vi "JSON Formater.vi"(4 "Disable LabVIEW Extensions":bool, 6 "Pretty Print":bool, 7 "Comment out unparsable lines":bool, 8 "error in":errorcluster, 10 "Offset":i32, 11 "JSON":string) -> (0 "error OUT":errorcluster, 2 "Rest of Input String":string, 3 "<JSON>":string)   [LabVIEW 2020, in "JSONtext.lvlib"]
uses:
  <vilib>/JDP Science/JSONtext/JSONtext.lvlib
  <vilib>/JDP Science/JSONtext/Parsing/Parsing State.ctl
  <vilib>/JDP Science/JSONtext/Parsing/Token Type.ctl
panel:
  in  "Pretty Print Levels":i32=9
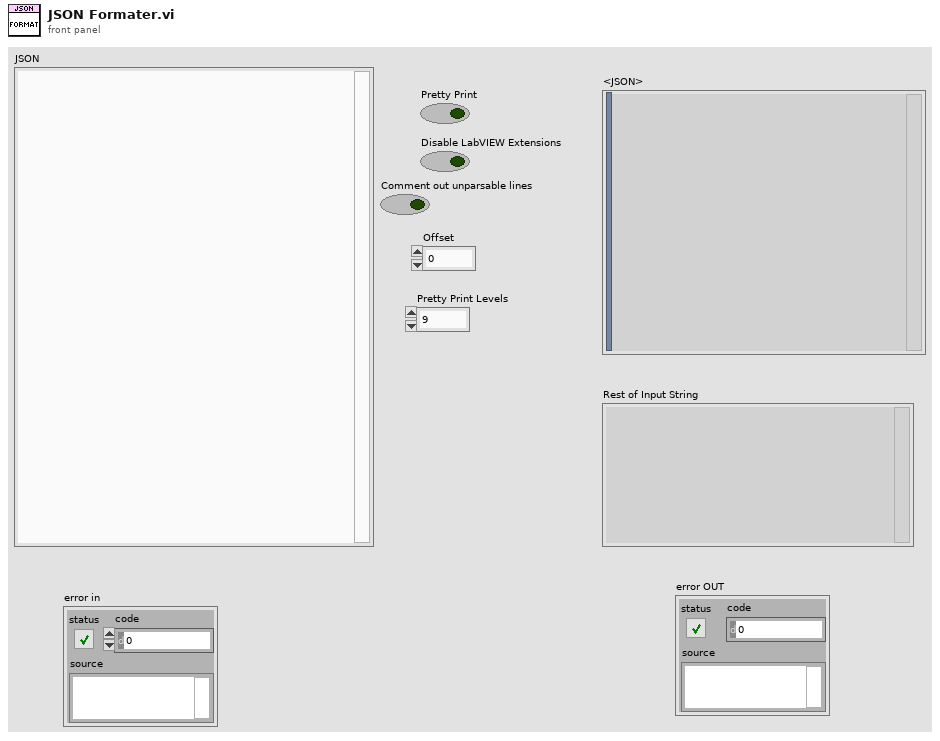
[diagram p1: front panel]
types:
  T1 = typedef "JSONtext.lvlib/Parsing State.ctl" = enum16{"Parser Error", "Object", "Array", "String", "Number/Other", "Leading Whitespace", "Object end", "Array end", "Value end"}
  T2 = typedef "JSONtext.lvlib/Token Type.ctl" = enum16{"Error", "Scalar", "comma", "colon", "Comment", "Down", "Up", "Line End", "Make Null", "Inline Comment", "Ignore", "junk line"}
  T3 = cluster{"Offset of first non-whitespace":i32, "Offset of first non-whitespace":i32, T2}
  T4 = typedef "JSONtext.lvlib/Token.ctl" = cluster{"Start":i32, "End":i32, "Type":T2}
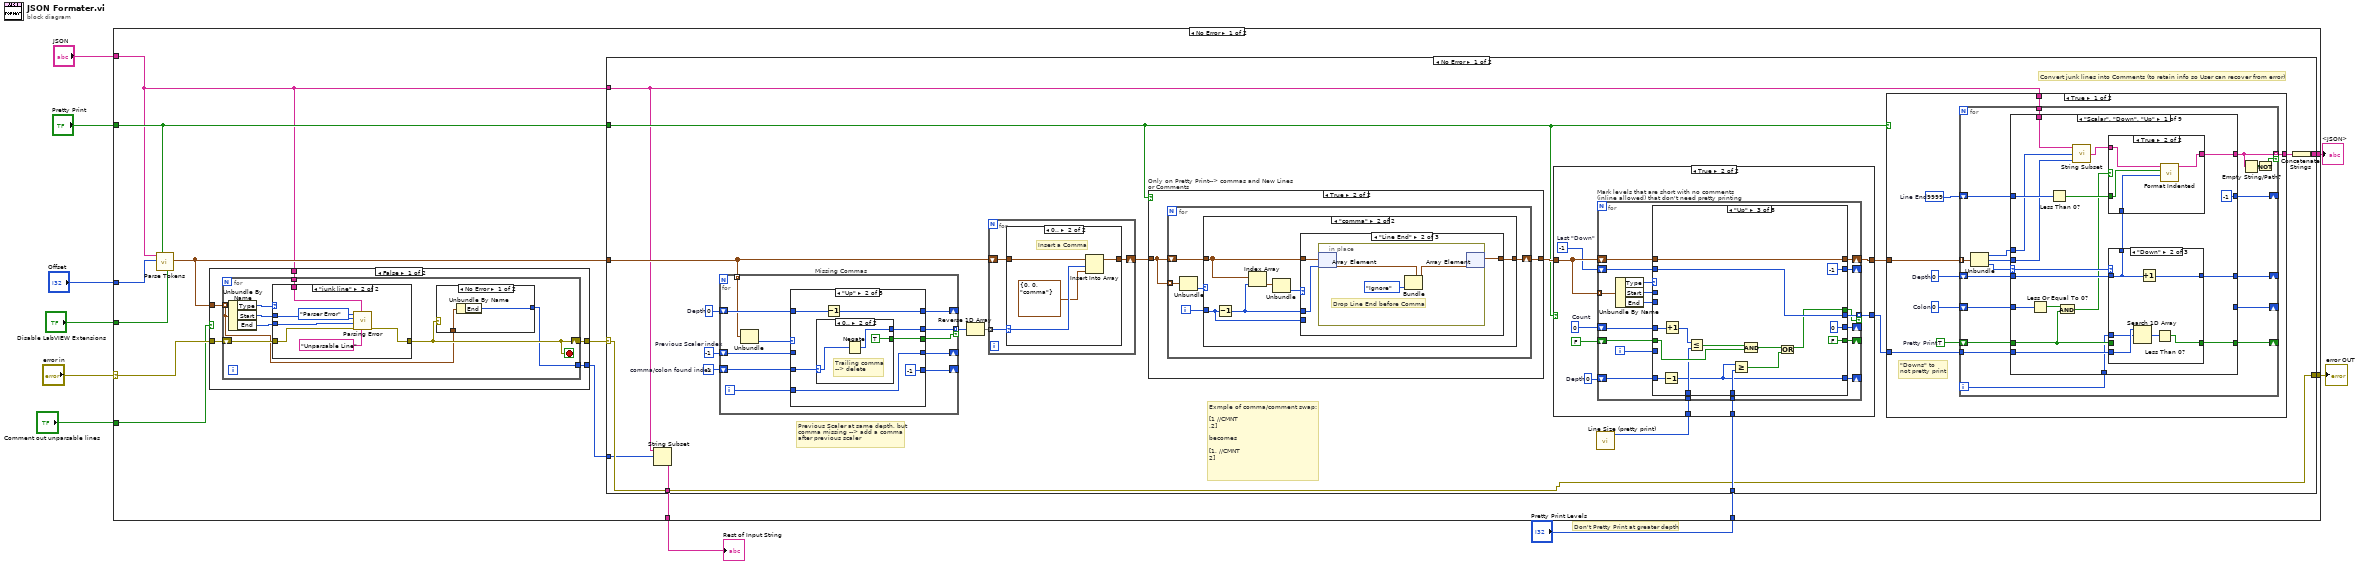
[diagram p0: block diagram]
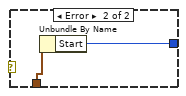
[diagram p2: hidden frame]
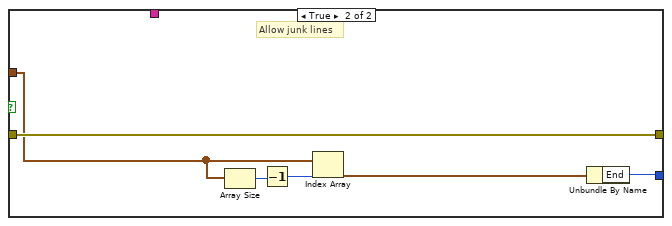
[diagram p4: hidden frame]
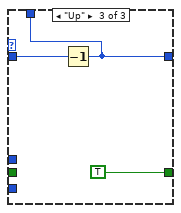
[diagram p7: hidden frame]
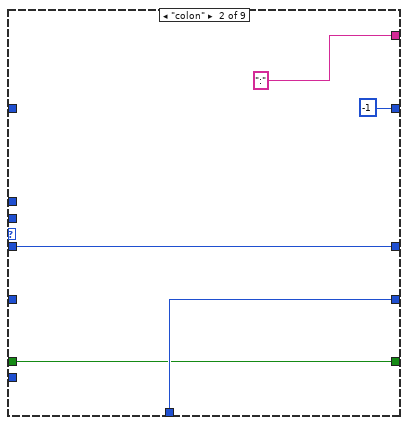
[diagram p8: hidden frame]
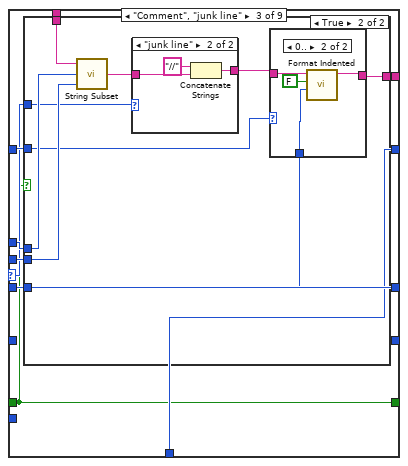
[diagram p9: hidden frame]
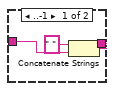
[diagram p12: hidden frame]
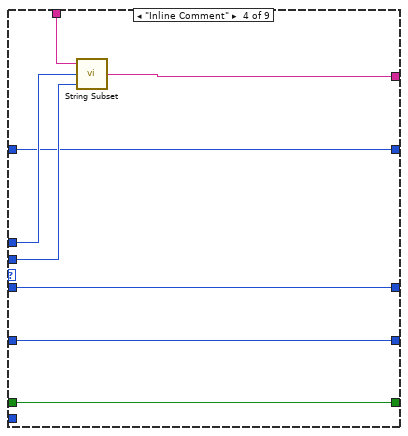
[diagram p13: hidden frame]
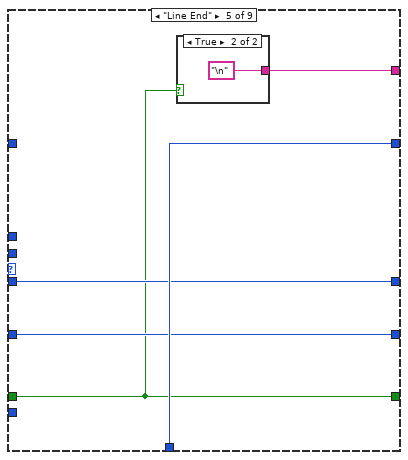
[diagram p14: hidden frame]
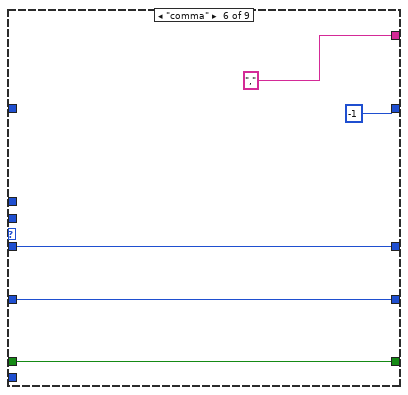
[diagram p16: hidden frame]
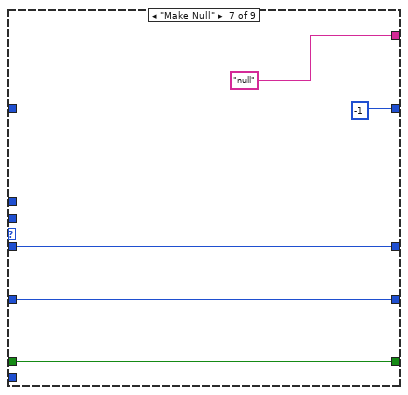
[diagram p17: hidden frame]
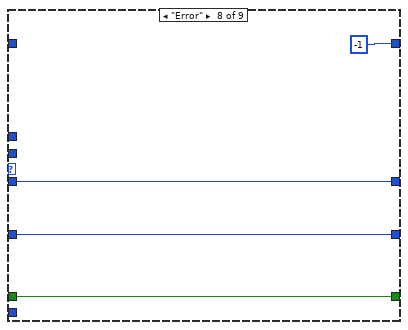
[diagram p18: hidden frame]
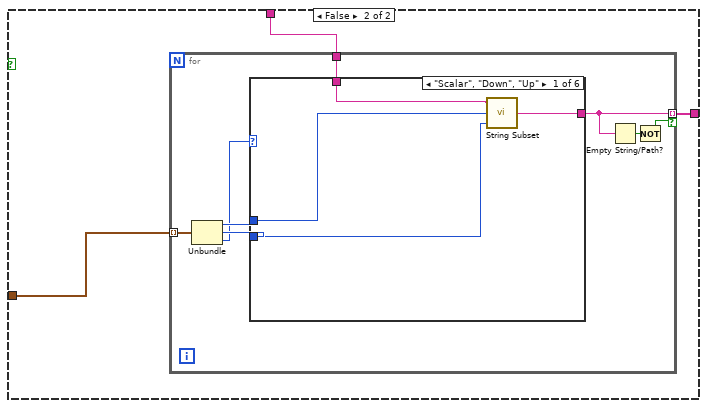
[diagram p20: hidden frame]
diagram:
  # "Don't Pretty Print at greater depth"
  n1 = case shown="No Error" "error in" {
    selector: "error in" -> [w18 w394]
    tunnel: [w23 _] -> w10
    tunnel: "Disable LabVIEW Extensions" -> [w22 _]
    tunnel: "Offset" -> [w21 _]
    tunnel: "Pretty Print" -> [w20 _]
    tunnel: "JSON" -> [w13 w393]
    tunnel: "Pretty Print Levels" -> [w17 _]
    tunnel: [w15 w394] -> w3
    tunnel: "Comment out unparsable lines" -> [w14 _]
    tunnel: [w11 w393] -> w1
    frame No Error {
      n2 = call <vilib>:"Parse Tokens.vi"("Disable LabVIEW Extensions"=w22, "Pretty Print"=w20, "Offset"=w21, "JSON"=w13) -> ("Tokens"=w19:T4[])  [unwired: 7 in]
      n3 = case shown="False" w14 {
        tunnel: w19 -> [w28 w53]
        tunnel: w13 -> [w27 _]
        tunnel: w18 -> [w26 w54]
        tunnel: [w25 w54] -> w16
        tunnel: [w24 w49] -> w12
        frame False {
          n4 = for {
            tunnel: w28 -> [w30] mode=indexing
            tunnel: w27 -> [w35]
            shift-right: [w31] -> w25
            shift-left: w26 -> [w34]
            tunnel: [w29] -> w24
            stop <- w31 stop-if-true
            n5 = Unbundle By Name(w30) -> ("Type"=w36:T2, "Start"=w32:i32, "End"=w33:i32)
            n6 = case shown="\"junk line\"" w36 {
              tunnel: w32 -> [_ w48]
              tunnel: w33 -> [_ w47]
              tunnel: w35 -> [_ w46]
              tunnel: w34 -> [w41 w43]
              tunnel: [w41 w42] -> w31
              frame "Error", Default {
              }
              frame "junk line" {
                n7 = call <vilib>:"Parsing Error.vi"("initial string"="Unparsable Line", "JSON"=w46, "error in (no error)"=w43, "Offset past match"=w47, "Value start"=w48, "State"=Parsing_State."Parser Error") -> ("error out"=w42:errorcluster)  [unwired: 5 in]
              }
            }
            n8 = case shown="No Error" w31 {
              tunnel: w30 -> [w38 w40]
              tunnel: [w37 w39] -> w29
              frame No Error {
                n9 = Unbundle By Name(w38) -> ("End"=w37:i32)
              }
              frame Error {
                n10 = Unbundle By Name(w40) -> ("Start"=w39:i32)
              }
            }
          }
        }
        frame True {
          # "Allow junk lines"
          n11 = Array Size(array=w53) -> (size(s)=w52:i32)
          n12 = Decrement(x=w52) -> (x-1=w51:i32)
          n13 = Index Array(array=w53, index=w51) -> (element=w50:T4)
          n14 = Unbundle By Name(w50) -> ("End"=w49:i32)
        }
      }
      n15 = case shown="No Error" w16 {
        selector: w16 -> [w58 w392]
        tunnel: [w72 _] -> w23
        tunnel: w20 -> [w64 _]
        tunnel: w19 -> [w60 _]
        tunnel: w13 -> [w57 w391]
        tunnel: w17 -> [w59 _]
        tunnel: [w58 w392] -> w15
        tunnel: w12 -> [w56 _]
        tunnel: [w55 w391] -> w11
        frame No Error {
          w69 = -1  # comma/colon found index
          w70 = -1  # Previous Scaler index
          w71 = 0  # Depth
          # "Exmple of comma/comment swap:\n\n[1 //CMNT\n,2]\n\nbecomes\n\n[1, //CMNT\n2]"
          # "Convert junk lines into Comments (to retain info so User can recover from error)"
          # "Previous Scaler at same depth, but\ncomma missing --> add a comma\nafter previous scaler"
          n16 = String Subset(string=w57, offset (0)=w56) -> (substring=w55:string)  [unwired: 1 in]
          n17 = for "Missing Commas" {
            shift-right: [w355] -> _
            shift-left: w71 -> [w356]
            shift-right: [w353] -> _
            shift-left: w70 -> [w354]
            shift-right: [w352] -> _
            shift-left: w69 -> [w351]
            tunnel: [w350] -> w68 mode=indexing if=w349
            tunnel: w60 -> [w347] mode=indexing
            i -> [w348]
            n18 = Unbundle(w347) -> ("Type"=w346:T2)  [unwired: 2 out]
            n19 = case shown="\"Up\"" w346 {
              tunnel: w356 -> [w359 w366 w375 w385 w389]
              tunnel: [w359 w365 w375 w380 w389] -> w355
              tunnel: w354 -> [w358 _ w373 w384 w390]
              tunnel: [w358 w360 w376 w379 w390] -> w353
              tunnel: [w357 -1 ("comma found index") -1 ("comma found index") w379 w388] -> w352
              tunnel: w351 -> [w357 w364 w378 w387 _]
              tunnel: [_ w363 w370 w381 _] -> w350
              tunnel: [_ w362 w372 w383 _] -> w349
              tunnel: w348 -> [_ w360 w376 _ w388]
              frame Default {
              }
              frame "Up" {
                n20 = case shown="0.." w364 {
                  selector: w364 -> [_ w369]
                  tunnel: [_ w368] -> w363
                  tunnel: [_ TRUE] -> w362
                  frame ..-1 {
                  }
                  frame 0.. {
                    # "Trailing comma\n--> delete"
                    n21 = Negate(x=w369) -> (-x=w368:i32)
                  }
                }
                n22 = Decrement(x=w366) -> (x-1=w365:i32)
              }
              frame "Scalar", "Make Null" {
                n23 = Greater Or Equal To 0?(x=w373) -> (x >= 0?=w371:bool)
                n24 = Less Than 0?(x=w378) -> (x < 0?=w377:bool)
                n25 = And(x=w371, y=w377) -> (x .and. y?=w372:bool)
                n26 = Increment(x=w373) -> (x+1=w370:i32)
              }
              frame "Down" {
                w379 = -1 ("comma found index")
                n27 = Greater Or Equal To 0?(x=w384) -> (x >= 0?=w382:bool)
                n28 = Less Than 0?(x=w387) -> (x < 0?=w386:bool)
                n29 = Increment(x=w385) -> (x+1=w380:i32)
                n30 = And(x=w382, y=w386) -> (x .and. y?=w383:bool)
                n31 = Increment(x=w384) -> (x+1=w381:i32)
              }
              frame "comma", "colon" {
              }
            }
          }
          n32 = Reverse 1D Array(array=w68) -> (reversed array=w67:i32[])
          n33 = for {
            tunnel: w67 -> [w309] mode=indexing
            shift-right: [w308] -> w66
            shift-left: w60 -> [w307]
            n34 = case shown="0.." w309 {
              selector: w309 -> [w311 w315]
              tunnel: [w312 w316] -> w308
              tunnel: w307 -> [w313 w317]
              frame ..-1 {
                # "Negative means delete a comma"
                n35 = Absolute Value(x=w311) -> (abs(x)=w310:i32)
                n36 = Delete From Array(array=w313, index=w310) -> (array with subset deleted=w312:T4[])  [unwired: 1 in, 1 out]
              }
              frame 0.. {
                # "Insert a Comma"
                n37 = Insert Into Array(array=w317, index=w315, new element=T3 {"Offset of first non-whitespace"=0, "Offset of first non-whitespace"=0, enum."comma"} ("new element/subarray")) -> (w316:T4[])
              }
            }
          }
          n38 = case "Only on Pretty Print--> commas and New Lines or Comments" shown="True" w64 {
            tunnel: w66 -> [w318 w320]
            tunnel: [w318 w319] -> w65
            frame False {
            }
            frame True {
              n39 = for {
                tunnel: w320 -> [w322] mode=indexing
                shift-right: [w321] -> w319
                shift-left: w320 -> [w324]
                i -> [w323]
                n40 = Unbundle(w322) -> ("Type"=w325:T2)  [unwired: 2 out]
                n41 = case shown="\"comma\"" w325 {
                  tunnel: w324 -> [w326 w330]
                  tunnel: w323 -> [_ w327]
                  tunnel: [w326 w329] -> w321
                  frame Default {
                  }
                  frame "comma" {
                    n42 = Decrement(x=w327) -> (x-1=w328:i32)
                    n43 = Index Array(array=w330, index=w328) -> (element=w332:T4)
                    n44 = Unbundle(w332) -> ("Type"=w331:T2)  [unwired: 2 out]
                    n45 = case shown="\"Line End\"" w331 {
                      tunnel: w330 -> [w333 w336 w343]
                      tunnel: [w333 w334 w341] -> w329
                      tunnel: w328 -> [_ w335 w342]
                      tunnel: w327 -> [_ _ w340]
                      frame Default {
                      }
                      frame "Line End" {
                        n46 = in-place {
                          # "Drop Line End before Comma"
                          n47 = in-place-array #1(w336, w335) -> (w339:T4)
                          n48 = Bundle(cluster=w339, "Type"=Token_Type."Ignore") -> (w338:T4)  [unwired: 2 in]
                          n49 = in-place-array #1(w338) -> (w334:T4[])  [unwired: 1 out]
                        }
                      }
                      frame "Comment" {
                        n50 = in-place {
                          # "Move Comma in front of precceding comment"
                          n51 = in-place-array #2(w343, w342, w340) -> (w345:T4, w344:T4)
                          n52 = in-place-array #2(w344, w345) -> (w341:T4[])  [unwired: 2 out]
                        }
                      }
                    }
                  }
                }
              }
            }
          }
          n53 = call <vilib>:"Line Size (pretty print).vi"() -> ("Line Size"=w61:i32)  [unwired: 11 in]
          n54 = case shown="True" w64 {
            tunnel: w65 -> [w219 w228]
            tunnel: [w219 w224] -> w63
            tunnel: [_ w223] -> w62
            tunnel: w61 -> [_ w222]
            tunnel: w59 -> [_ w221]
            frame False {
            }
            frame True {
              w220 = 0  # Depth
              w225 = -1  # Last "Down"
              w227 = 0  # Count
              n55 = for "Mark levels that are short with no comments (inline allowed) that don't need pretty printing" {
                tunnel: w228 -> [w247] mode=indexing
                shift-right: [w244] -> w224
                shift-left: w228 -> [w245]
                shift-right: [w240] -> _
                shift-left: w227 -> [w241]
                shift-right: [w239] -> _
                shift-left: FALSE -> [w238]
                shift-right: [w236] -> _
                shift-left: w225 -> [w237]
                tunnel: [w234] -> w223 mode=indexing if=w233
                tunnel: w222 -> [w232]
                tunnel: w221 -> [w231]
                shift-right: [w229] -> _
                shift-left: w220 -> [w230]
                i -> [w235]
                n56 = Unbundle By Name(w247) -> ("Type"=w246:T2, "Start"=w243:i32, "End"=w242:i32)
                n57 = case shown="\"Up\"" w246 {
                  tunnel: w245 -> [w252 w258 w270 w279 w286 w292 w301 w306]
                  tunnel: [w252 w258 w270 w279 w286 w292 w301 w306] -> w244
                  tunnel: w243 -> [_ _ _ _ _ _ w299 _]
                  tunnel: w242 -> [_ _ _ _ _ _ w300 _]
                  tunnel: w241 -> [w250 _ w264 w278 w285 w291 w298 w305]
                  tunnel: [w250 1 0 ("count") w278 w283 w289 w296 w305] -> w240
                  tunnel: [w251 TRUE FALSE w277 w284 w290 w295 FALSE] -> w239
                  tunnel: w238 -> [w251 _ w268 w277 w284 w290 w295 _]
                  tunnel: w237 -> [w249 _ w267 w276 w281 w288 w294 w303]
                  tunnel: [w249 w255 -1 ("Last Down") w276 w281 w288 w294 w303] -> w236
                  tunnel: w235 -> [_ w255 _ _ _ _ _ _]
                  tunnel: [_ _ w267 _ _ _ _ _] -> w234
                  tunnel: [_ _ w260 _ _ _ _ _] -> w233
                  tunnel: w232 -> [_ _ w265 _ _ _ _ _]
                  tunnel: w231 -> [_ _ w263 _ _ _ _ _]
                  tunnel: w230 -> [w248 w254 w262 w275 w280 w287 w293 w302]
                  tunnel: [w248 w253 w261 w275 w280 w287 w293 w302] -> w229
                  frame "Error" {
                  }
                  frame "Down" {
                    n58 = Increment(x=w254) -> (x+1=w253:i32)
                  }
                  frame "Up" {
                    n59 = Decrement(x=w262) -> (x-1=w261:i32)
                    n60 = Increment(x=w264) -> (x+1=w272:i32)
                    n61 = Less Or Equal?(x=w272, y=w265) -> (x <= y?=w269:bool)
                    n62 = Greater Or Equal?(x=w261, y=w263) -> (x >= y?=w259:bool)
                    n63 = Compound Arithmetic op=AND(w269, w268) -> (w266:bool)
                    n64 = Or(x=w266, y=w259) -> (x .or. y?=w260:bool)
                  }
                  frame "Line End", "Ignore" {
                  }
                  frame "Make Null" {
                    n65 = Add(x=w285, y=4) -> (x+y=w283:i32)
                  }
                  frame "comma", "colon" {
                    n66 = Increment(x=w291) -> (x+1=w289:i32)
                  }
                  frame "Scalar", "Inline Comment" {
                    n67 = Subtract(x=w300, y=w299) -> (x-y=w297:i32)
                    n68 = Add(x=w298, y=w297) -> (x+y=w296:i32)
                  }
                  frame "Comment", "junk line" {
                  }
                }
              }
            }
          }
          n69 = case shown="True" w64 {
            tunnel: w57 -> [w81 w203]
            tunnel: [w80 w202] -> w73
            tunnel: w63 -> [w79 w201]
            tunnel: w62 -> [w75 _]
            frame True {
              w74 = TRUE  # Pretty Print
              w76 = 0  # Colon
              w77 = 0  # Depth
              w78 = 9999  # Line End
              # "\"Downs\" to \nnot pretty print"
              n70 = for {
                tunnel: w79 -> [w99] mode=indexing
                tunnel: w81 -> [w98]
                tunnel: [w97] -> w80 mode=indexing if=w95
                shift-right: [w94] -> _
                shift-left: w78 -> [w92]
                shift-right: [w90] -> _
                shift-left: w77 -> [w91]
                shift-right: [w88] -> _
                shift-left: w76 -> [w89]
                tunnel: w75 -> [w84]
                shift-right: [w83] -> _
                shift-left: w74 -> [w82]
                i -> [w93]
                n71 = Unbundle(w99) -> ("Start"=w87:i32, "End"=w86:i32, "Type"=w85:T2)
                n72 = case shown="\"Scalar\", \"Down\", \"Up\"" w85 {
                  selector: w85 -> [w113 _ w141 _ _ _ _ _ _]
                  tunnel: w98 -> [w118 _ w148 w176 _ _ _ _ _]
                  tunnel: [w116 ":" ("substring") w145 w170 w181 "," ("substring") "null" ("substring") _ _] -> w97
                  tunnel: [-1 ("Line End") -1 ("Line End") w143 w171 w180 -1 ("Line End") -1 ("Line End") -1 ("Line End") w198] -> w94
                  tunnel: w93 -> [w100 w137 w143 _ w180 _ _ _ _]
                  tunnel: w92 -> [w117 _ w142 w171 _ _ _ _ w198]
                  tunnel: w91 -> [w112 w138 w144 w173 w179 w186 w191 w196 w200]
                  tunnel: [w114 w138 w144 w173 w179 w186 w191 w196 w200] -> w90
                  tunnel: w89 -> [w110 _ _ w172 w178 w185 w190 w195 w199]
                  tunnel: [_ w137 _ w172 w178 w185 w190 w195 w199] -> w88
                  tunnel: w87 -> [w108 _ w147 w175 _ _ _ _ _]
                  tunnel: w86 -> [w107 _ w146 w174 _ _ _ _ _]
                  tunnel: w84 -> [w105 _ _ _ _ _ _ _ _]
                  tunnel: [w104 w135 w140 w169 w177 w183 w188 w193 w197] -> w83
                  tunnel: w82 -> [w101 w135 w140 w169 w177 w183 w188 w193 w197]
                  frame "Scalar", "Down", "Up" {
                    n73 = Less Or Equal To 0?(x=w110) -> (x <= 0?=w103:bool)
                    n74 = Less Than 0?(x=w117) -> (x < 0?=w115:bool)
                    n75 = And(x=w103, y=w101) -> (x .and. y?=w102:bool)
                    n76 = call <vilib>:"String Subset.vi"("Offset past End"=w107, "Start offset"=w108, "JSON"=w118) -> ("substring"=w109:string)  [unwired: 2 in]
                    n77 = case shown="\"Down\"" w113 {
                      tunnel: w112 -> [w125 w130 w134]
                      tunnel: [w125 w131 w133] -> w114
                      tunnel: [w125 w130 w133] -> w111
                      tunnel: w105 -> [_ w129 _]
                      tunnel: [w124 w126 TRUE ("Pretty Print")] -> w104
                      tunnel: w101 -> [w124 _ _]
                      tunnel: w100 -> [_ w128 _]
                      frame Default {
                      }
                      frame "Down" {
                        n78 = Search 1D Array(1D array=w129, element=w128) -> (index of element=w127:i32)  [unwired: 1 in]
                        n79 = Increment(x=w130) -> (x+1=w131:i32)
                        n80 = Less Than 0?(x=w127) -> (x < 0?=w126:bool)
                      }
                      frame "Up" {
                        n81 = Decrement(x=w134) -> (x-1=w133:i32)
                      }
                    }
                    n82 = case shown="True" w102 {
                      tunnel: [w119 w123] -> w116
                      tunnel: w115 -> [_ w122]
                      tunnel: w111 -> [_ w121]
                      tunnel: w109 -> [w119 w120]
                      frame False {
                      }
                      frame True {
                        n83 = call <vilib>:"Format Indented.vi"("Depth"=w121, "New Line needed"=w122, "Text"=w120) -> ("Indented Text"=w123:string)  [unwired: 8 in]
                      }
                    }
                  }
                  frame "colon" {
                  }
                  frame "Comment", "junk line" {
                    n84 = case shown="True" w140 {
                      tunnel: w148 -> [_ w157]
                      tunnel: w147 -> [_ w156]
                      tunnel: w146 -> [_ w155]
                      tunnel: [_ w153] -> w145
                      tunnel: w144 -> [_ w152]
                      tunnel: w142 -> [_ w151]
                      tunnel: w141 -> [_ w149]
                      frame False {
                      }
                      frame True {
                        n85 = call <vilib>:"String Subset.vi"("Offset past End"=w155, "Start offset"=w156, "JSON"=w157) -> ("substring"=w154:string)  [unwired: 2 in]
                        n86 = case shown="\"junk line\"" w149 {
                          tunnel: w154 -> [w158 w161]
                          tunnel: [w158 w160] -> w150
                          frame Default {
                          }
                          frame "junk line" {
                            n87 = Concatenate Strings("//" ("string"), w161) -> (w160:string)
                          }
                        }
                        n88 = case shown="0.." w151 {
                          tunnel: [w163 w167] -> w153
                          tunnel: w152 -> [_ w165]
                          tunnel: w150 -> [w164 w168]
                          frame ..-1 {
                            n89 = Concatenate Strings(" " ("string"), w164) -> (w163:string)
                          }
                          frame 0.. {
                            n90 = call <vilib>:"Format Indented.vi"("Depth"=w165, "New Line needed"=FALSE, "Text"=w168) -> ("Indented Text"=w167:string)  [unwired: 8 in]
                          }
                        }
                      }
                    }
                  }
                  frame "Inline Comment" {
                    n91 = call <vilib>:"String Subset.vi"("Offset past End"=w174, "Start offset"=w175, "JSON"=w176) -> ("substring"=w170:string)  [unwired: 2 in]
                  }
                  frame "Line End" {
                    n92 = case shown="True" w177 {
                      tunnel: [_ "\n" ("substring")] -> w181
                      frame False {
                      }
                      frame True {
                      }
                    }
                  }
                  frame "comma" {
                  }
                  frame "Make Null" {
                  }
                  frame "Error" {
                  }
                  frame "Ignore" {
                  }
                }
                n93 = Empty String/Path?(string/path=w97) -> (empty?=w96:bool)
                n94 = Not(x=w96) -> (.not. x?=w95:bool)
              }
            }
            frame False {
              n95 = for {
                tunnel: w201 -> [w211] mode=indexing
                tunnel: w203 -> [w210]
                tunnel: [w209] -> w202 mode=indexing if=w207
                n96 = Unbundle(w211) -> ("Start"=w206:i32, "End"=w205:i32, "Type"=w204:T2)
                n97 = case shown="\"Scalar\", \"Down\", \"Up\"" w204 {
                  tunnel: w210 -> [w215 _ _ _ _ _]
                  tunnel: [w214 "," ("substring") ":" ("substring") "null" ("substring") _ _] -> w209
                  tunnel: w206 -> [w213 _ _ _ _ _]
                  tunnel: w205 -> [w212 _ _ _ _ _]
                  frame "Scalar", "Down", "Up" {
                    n98 = call <vilib>:"String Subset.vi"("Offset past End"=w212, "Start offset"=w213, "JSON"=w215) -> ("substring"=w214:string)  [unwired: 2 in]
                  }
                  frame "comma" {
                  }
                  frame "colon" {
                  }
                  frame "Make Null" {
                  }
                  frame Default {
                  }
                  frame "Error" {
                  }
                }
                n99 = Empty String/Path?(string/path=w209) -> (empty?=w208:bool)
                n100 = Not(x=w208) -> (.not. x?=w207:bool)
              }
            }
          }
          n101 = Concatenate Strings(w73) -> (w72:string)
        }
        frame Error {
        }
      }
    }
    frame Error {
    }
  }
  "<JSON>" <- w10
  "error OUT" <- w3
  "Rest of Input String" <- w1
